vi "test Cluster Handles.vi"(8 "error in (no error)":errorcluster, 11 "TestCase in":refnum<class "Data Structure Tests.lvclass">) -> (0 "error out":errorcluster, 3 "TestCase out":refnum<class "Data Structure Tests.lvclass">)   [LabVIEW 2020, in "Data Structure Tests.lvclass"]
uses:
  Data Structure Tests.lvclass
  Data Structure Tests.lvclass/Data Structure Tests.ctl
  <vilib>/addons/_JKI Toolkits/VI Tester/TestCase.llb/TestCase.lvclass
  C:/Program Files (x86)/National Instruments/LabVIEW 2020/vi.lib/addons/_JKI Toolkits/VI Tester/TestCase.llb/TestCase.lvclass
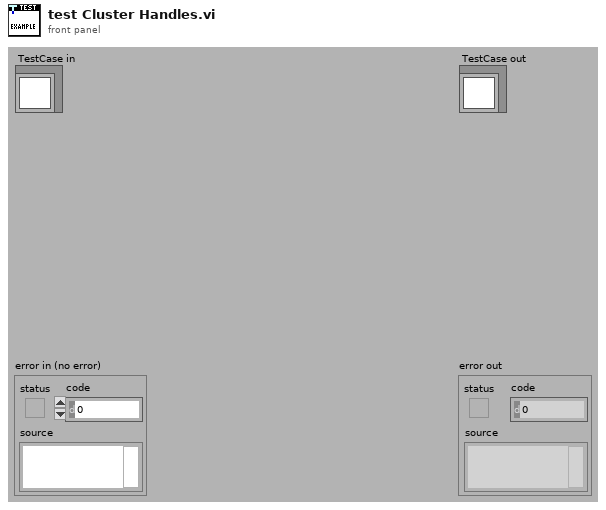
[diagram p1: front panel]
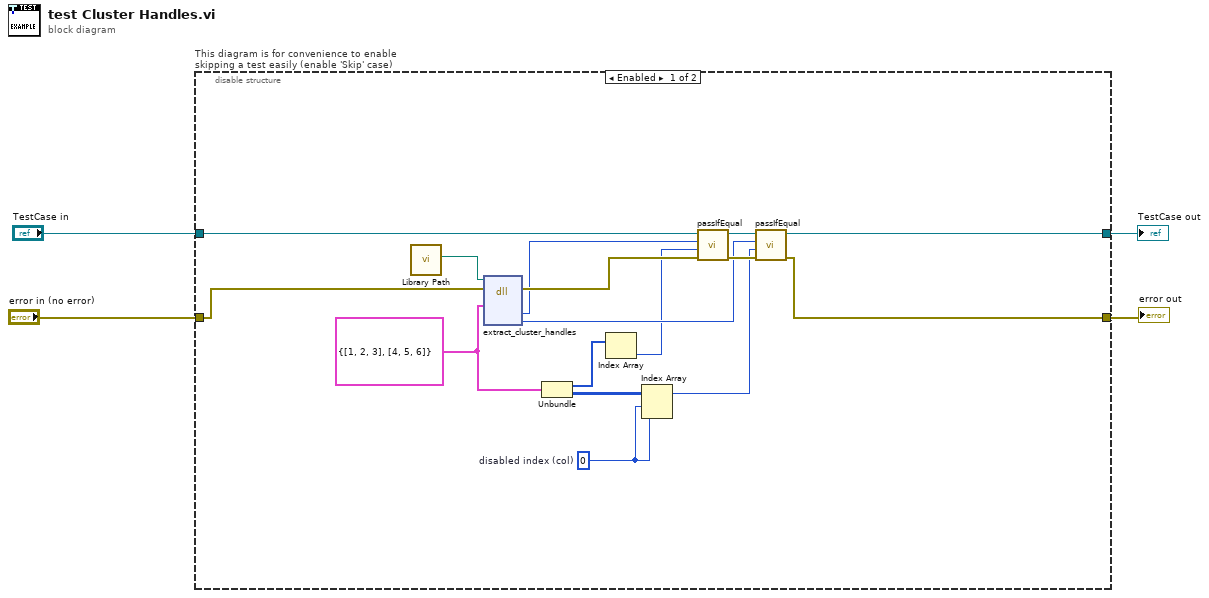
[diagram p0: block diagram]
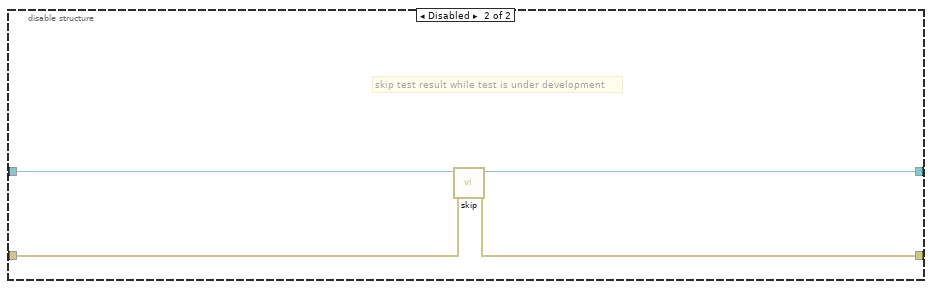
[diagram p2: hidden frame]
diagram:
  n1 = disable-structure "This diagram is for convenience to enable skipping a test easily (enable 'Skip' case)" shown="Enabled" {
    disable-tunnel: "TestCase in" -> [w20 w24]
    disable-tunnel: [w14 w22] -> w1
    disable-tunnel: [w16 w23] -> w3
    disable-tunnel: "error in (no error)" -> [w18 w21]
    frame Enabled {
      w6 = 0  # disabled index (col)
      w11 = cluster{u8[], u32[][]} {[1, 2, 3], [[4, 5, 6]]}
      n2 = call "Library Path.vi"() -> ("Library Path"=w5:path)  [unwired: 11 in]
      n3 = dll-call lib="C:/Users/JamesMcNally/Documents/RustInterop/Rust-LabVIEW-Interop/target/debug/labview_test_library.dll" fn="extract_cluster_handles"(path in=w5, error in=w18, "struct"=w11) -> (error out=w17:errorcluster, "one"=w13:u8, "two"=w12:u32)  [unwired: 5 in, 1 out]
      n4 = Unbundle(w11) -> (w10:u8[], w9:u32[][])
      n5 = Index Array(array=w10) -> (element=w8:u8)  [unwired: 1 in]
      n6 = Index Array(array=w9, index (row)=w6, index (col)=w6) -> (element=w7:u32)
      n7 = call-dynamic "passIfEqual.vi"("error in (no error)"=w17, "y"=w8, "x"=w13, "TestCase in"=w20) -> ("error out"=w19:errorcluster, "TestCase out"=w15:refnum<class "Data Structure Tests.lvclass">)  [unwired: 6 in]
      n8 = call-dynamic "passIfEqual.vi"("error in (no error)"=w19, "y"=w7, "x"=w12, "TestCase in"=w15) -> ("error out"=w16:errorcluster, "TestCase out"=w14:refnum<class "Data Structure Tests.lvclass">)  [unwired: 6 in]
    }
    frame Disabled {
      # "skip test result while test is under development"
      n9 = call <vilib>:"skip.vi"("error in (no error)"=w21, "TestCase in"=w24) -> ("error out"=w23:errorcluster, "TestCase out"=w22:refnum<class "Data Structure Tests.lvclass">)  [unwired: 8 in]
    }
  }
  "error out" <- w3
  "TestCase out" <- w1
